vi "Paths to String with Commas.vi"(10 "Array":string[](array[string])) -> (1 "Columns":string, 2 "Table":string)   [LabVIEW 2020, in "Data.PG.lvclass"]
uses:
  Data.PG.lvclass
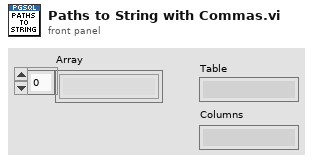
[diagram p1: front panel]
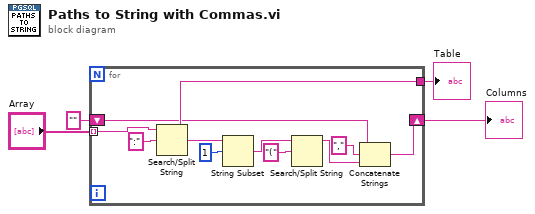
[diagram p0: block diagram]
diagram:
  n1 = for {
    shift-right: [w12] -> w4
    shift-left: "" -> [w6]
    tunnel: [w11] -> w3
    tunnel: "Array" -> [w5] mode=indexing
    n2 = Search/Split String(string=w5, search string/char (-)=":") -> (substring before match=w11:string, match + rest of string=w14:string)  [unwired: 1 in, 1 out]
    n3 = String Subset(string=w14, offset (0)=1) -> (substring=w9:string)  [unwired: 1 in]
    n4 = Search/Split String(string=w9, search string/char (-)="(") -> (substring before match=w8:string)  [unwired: 1 in, 2 out]
    n5 = Concatenate Strings(w6, "," ("string"), w8) -> (w12:string)
  }
  "Columns" <- w4
  "Table" <- w3
